vi "Ej_12_DAQ_Lectura_Analogica.vi"() -> ()   [LabVIEW 2021]
panel:
  out "Salida Flip Flop":bool
  out "Salida":bool
  in  "Sensor":dbl
  in  "stop":bool
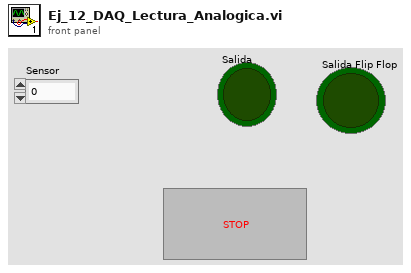
[diagram p1: front panel]
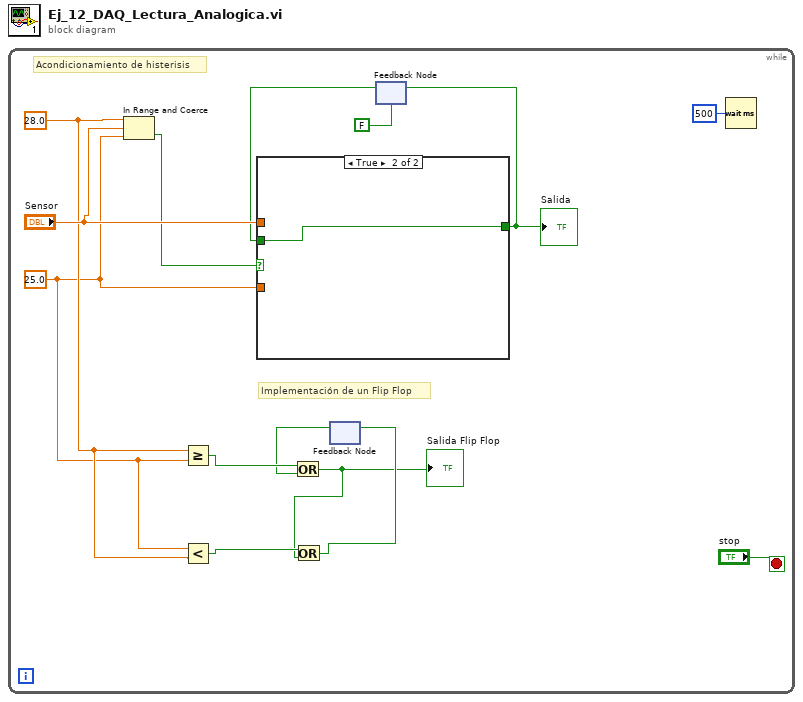
[diagram p0: block diagram]
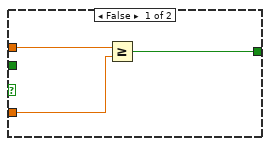
[diagram p2: hidden frame]
diagram:
  n1 = while {
    stop <- "stop" stop-if-true
    w6 = 25.0 ("lower limit")
    w7 = 28.0 ("upper limit")
    # "Implementación de un Flip Flop"
    # "Acondicionamiento de histerisis"
    n2 = In Range and Coerce(upper limit=w7, x="Sensor", lower limit=w6) -> (In Range?=w11:bool)  [unwired: 1 out]
    n3 = Greater Or Equal?(x=w7, y=w6) -> (x >= y?=w5:bool)
    n4 = Less?(x=w6, y=w7) -> (x < y?=w4:bool)
    n5 = feedback #1() -> (w2:bool)  [unwired: 1 in]
    n6 = Or(x=w5, y=w2) -> (x .or. y?=w1:bool)
    "Salida Flip Flop" <- w1
    n7 = Or(x=w4, y=w1) -> (x .or. y?=w3:bool)
    n8 = feedback-in #1(w3) -> ()
    n9 = feedback #2(FALSE) -> (w10:bool)
    n10 = case shown="True" w11 {
      tunnel: "Sensor" -> [w17 _]
      tunnel: w6 -> [w16 _]
      tunnel: [w15 w18] -> w9
      tunnel: w10 -> [_ w18]
      frame False {
        n11 = Greater Or Equal?(x=w17, y=w16) -> (x >= y?=w15:bool)
      }
      frame True {
      }
    }
    "Salida" <- w9
    n12 = feedback-in #2(w9) -> ()
    n13 = Wait (ms)(milliseconds to wait=u32 500) -> ()  [unwired: 1 out]
  }
